vi "Dataflow Example.vi"() -> ()   [LabVIEW 2010]
doc: "This VI demonstrates reading from and writing to a file. When this is not done in the proper order, the VI will give unexpected results."
uses:
  Type.ctl
panel:
  in  "File Entry":T2
  out "Updated Text":string
  out "Current Text":string
  in  "Save":bool
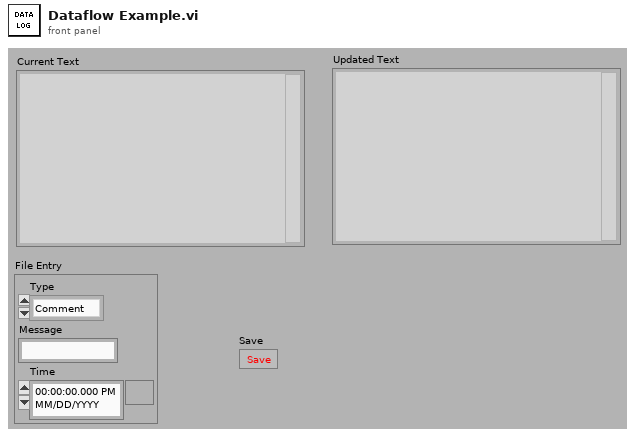
[diagram p1: front panel]
types:
  T1 = typedef "Type.ctl" = enum16{"Comment", "Question", "Concern"}
  T2 = cluster{"Type":T1, "Message":string, "Time":timestamp}
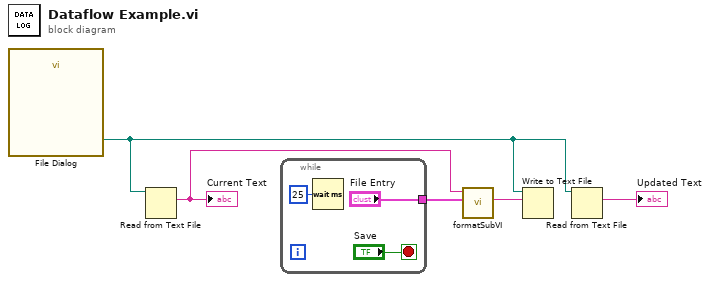
[diagram p0: block diagram]
diagram:
  n1 = call "File Dialog"() -> ("selected path"=w4:path)  [unwired: 12 in, 3 out]
  n2 = Read from Text File(file (use dialog)=w4) -> (text=w2:string)  [unwired: 3 in, 3 out]
  "Current Text" <- w2
  n3 = while {
    tunnel: ["File Entry"] -> w3
    stop <- "Save" stop-if-true
    n4 = Wait (ms)(milliseconds to wait=u32 25) -> ()  [unwired: 1 out]
  }
  n5 = call "formatSubVI.vi"("Message"=w3, "Current Text"=w2) -> ("Text Out"=w1:string)  [unwired: 7 in, 2 out]
  n6 = Write to Text File(file (use dialog)=w4, text=w1) -> ()  [unwired: 2 in, 3 out]
  n7 = Read from Text File(file (use dialog)=w4) -> (text=→"Updated Text":string)  [unwired: 3 in, 3 out]
